vi "Set Subpanel Visibility.vi"(8 "error in (no error)":errorcluster, 9 "Visible":bool, 10 "SubPanel":refnum<vi>, 11 "Manager in":refnum<class "Manager.lvclass">) -> (0 "error out":errorcluster, 3 "Manager out":refnum<class "Manager.lvclass">)   [LabVIEW 2020, in "OOPanel.lvlib" / "Manager.lvclass"]
doc: "Given a Subpanel reference, causes the panel contained in the subpanel to receive an event so it can update its state to the proper visibility. The visibility state of the subpanel will also be cached by the manager so panels will be signalled appropriately when being inserted while the subpanel is hidden.\n\nThis is useful for VIs containing managed subpanels being hidden and being able to forward that state appropriately to potentially nested panels. Another use-case is for subpanels in tab controls that can be told they're hidden whenever they're not the visible tab."
uses:
  Manager.lvclass
  Visibility State.ctl
  Manager.lvclass/Manager.ctl
  <vilib>/Utility/miscctls.llb/LVMapReplaceAction.ctl
  Panel/Panel.lvclass
  OOPanel.lvlib
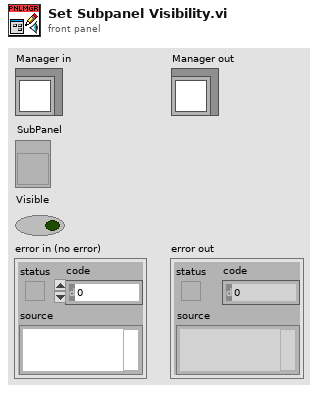
[diagram p1: front panel]
types:
  T1 = typedef "OOPanel.lvlib/Visibility State.ctl" = enum16{"Idle", "Closed", "Hidden", "Visible", "Subpanel", "Hidden Subpanel"}
  T2 = typedef "LVMapReplaceAction.ctl" = enum32{"Modify Entry only if found", "Add or Modify Entry", "Delete Entry"}
  T3 = typedef "OOPanel.lvlib/Manager.lvclass/Ref Data.ctl" = cluster{"Created Panels":refnum<class "Panel.lvclass">[], "Subpanel Map":map{refnum<vi>, T4}}
  T4 = typedef "OOPanel.lvlib/Manager.lvclass/Subpanel Data.ctl" = cluster{"Panel":refnum<class "Panel.lvclass">, "Has Panel":bool, "Visible":bool}
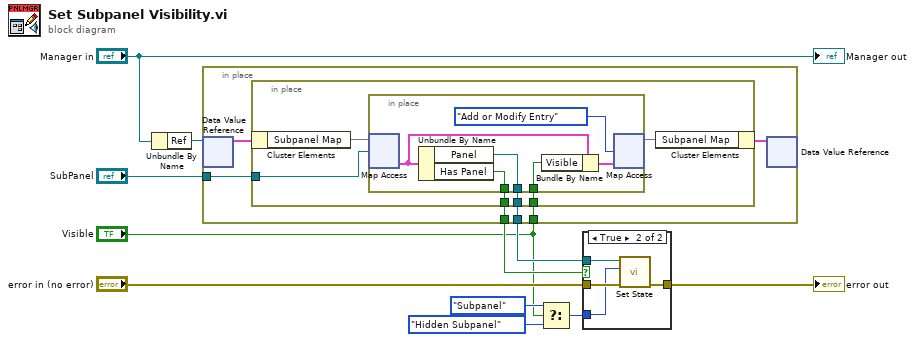
[diagram p0: block diagram]
diagram:
  n1 = Unbundle By Name("Manager in") -> ("Ref"=w11:refnum<data-value>)
  n2 = in-place {
    in-place-border: "SubPanel" -> [w15]
    in-place-border: [w14] -> w4
    in-place-border: [w13] -> w3
    in-place-border: "Visible" -> [w12]
    n3 = in-place-dvr #1(w11) -> (w17:T3)  [unwired: 1 out]
    n4 = in-place {
      in-place-border: w15 -> [w22]
      in-place-border: [w21] -> w14
      in-place-border: [w20] -> w13
      in-place-border: w12 -> [w19]
      n5 = in-place-cluster #2(w17) -> ("Subpanel Map"=w23:map{refnum<vi>, T4})
      n6 = in-place {
        in-place-border: [w26] -> w21
        in-place-border: [w25] -> w20
        in-place-border: w19 -> [w24]
        n7 = in-place-map #3(w23, w22) -> (w28:T4)  [unwired: 1 in, 1 out]
        n8 = Unbundle By Name(w28) -> ("Panel"=w25:refnum<class "Panel.lvclass">, "Has Panel"=w26:bool)
        n9 = Bundle By Name(cluster=w28, "Visible"=w24) -> (w27:T4)
        n10 = in-place-map #3(w27, LVMapReplaceAction."Add or Modify Entry" ("action")) -> (w18:map{refnum<vi>, T4})  [unwired: 2 out]
      }
      n11 = in-place-cluster #2("Subpanel Map"=w18) -> (w16:T3)
    }
    n12 = in-place-dvr #1(w16) -> ()  [unwired: 2 out]
  }
  n13 = Select(t=Visibility_State."Subpanel" ("State"), s="Visible", f=Visibility_State."Hidden Subpanel" ("State")) -> (s? t:f=w6:T1)
  n14 = case shown="True" w4 {
    tunnel: w3 -> [_ w34]
    tunnel: "error in (no error)" -> [w30 w33]
    tunnel: [w30 w32] -> w1
    tunnel: w6 -> [_ w31]
    frame False {
    }
    frame True {
      n15 = call "Set State.vi"("error in (no error)"=w33, "State"=w31, "Panel in"=w34) -> ("error out"=w32:errorcluster)  [unwired: 7 in, 1 out]
    }
  }
  "error out" <- w1
  "Manager out" <- "Manager in"
